vi "Start prototype.vi"() -> ()   [LabVIEW 2020]
panel:
  out "Waveform Graph":dbl[](graph)
  out "Waveform Chart":dbl(graph)
  out "Numeric":dbl
  in  "stop":bool
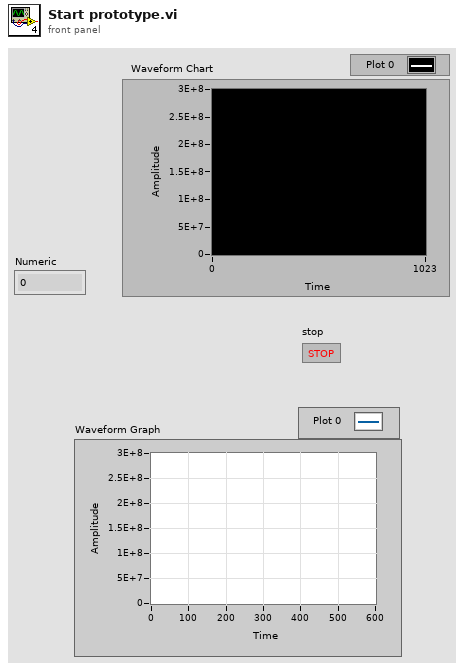
[diagram p1: front panel]
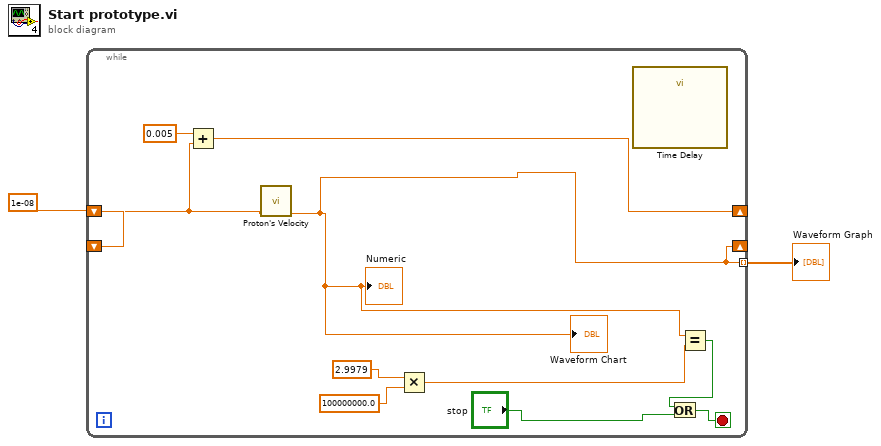
[diagram p0: block diagram]
diagram:
  w1 = 1e-08
  n1 = while {
    shift-right: [w7] -> _
    shift-left: w1 -> [w8]
    tunnel: [w6] -> w2 mode=indexing
    shift-right: [w6] -> _
    shift-left: w1 -> [_]
    stop <- w11 stop-if-true
    n2 = Add(x=0.005, y=w8) -> (x+y=w7:dbl)
    n3 = call "Proton's Velocity.vi"("Starting kinetic energy"=w8) -> ("Velocity (energy computed)"=w6:dbl)  [unwired: 9 in, 1 out]
    "Numeric" <- w6
    "Waveform Chart" <- w6
    n4 = Multiply(x=2.9979, y=100000000.0) -> (x*y=w3:dbl)
    n5 = call "Time Delay"() -> ()  [unwired: 11 in, 1 out]
    n6 = Equal?(x=w6, y=w3) -> (x = y?=w10:bool)
    n7 = Or(x=w10, y="stop") -> (x .or. y?=w11:bool)
  }
  "Waveform Graph" <- w2
